vi "LightStrip25.vi"() -> ()   [LabVIEW 2023]
uses:
  <vilib>/Platform/TimedLoop/XDataNode/timing_clust.ctl
  <vilib>/Platform/TimedLoop/XDataNode/nitl_modes.ctl
  <vilib>/Platform/TimedLoop/XDataNode/wakeup.ctl
  <vilib>/platform/TimedLoop/XDataNode/XDataNode.xnode
  <vilib>/Platform/TimedLoop/XDataNode/XDNodeRunTimeDep.lvlib
  BlingLibrary/ArduinoSerialBling.lvlib
panel:
  out "?":string
  in  "Driver color":u32(colorbox)
  in  "Match Ending \"timer\" (s)":dbl(slide) scale=0.0..30.0 scale format="%#_2g"
  in  "Robot State":T1(ring)
  out "LEDs":u32[](array[colorbox])
  in  "?":bool
  # "Light modes:\n\nConnected (default): \"pit mode\"; lights should be off by default during match\n\nDisconnected: flash red when disconnected/disabled?\n\nAutonomous: purple during auto\n\nAlgae: flash teal when running algae intake\n\nCoral: white when running coral intake\n\nOuttaking: flash green when outtaking/scoring\n\nAuto align; brief rainbow when aligning to Apriltag\n\nMatch ending: slowly slide timer to \"simulate\". Blue to red from outside, flash white when match end\n\nDefense: police strobe if/when defending\n\nDriver color: can be set on dashboard"
  # "Light strip"
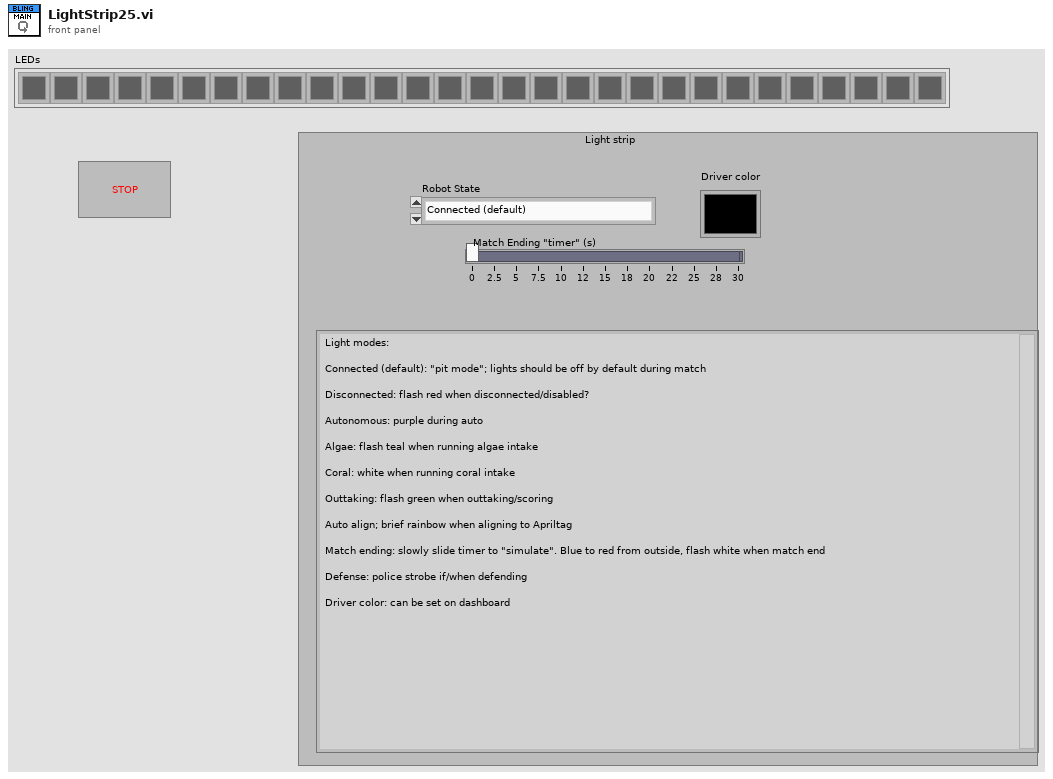
[diagram p1: front panel]
types:
  T1 = enum16{"Connected (default)", "Disconnected", "Autonomous", "Algae intake", "Coral intake", "Outtaking", "Auto align", "Match Ending", "Defense", "Driver Color"}
  T2 = enum16{"Connected (default)", "Disconnected", "Autonomous", "Browning", "Algae", "Coral", "Outtaking", "Auto align", "Match ending", "Defense", "Driver Color"}
  T3 = typedef "ArduinoSerialBling.lvlib/ControlState.ctl" = cluster{"VISA resource name":refnum<visa-resource-name>, "Synchronous":bool, "Value Width":enum16{"4-bit", "8-bit"}, "ChainMask":u8, "Chains":T4[], "OfflineMode":bool}
  T4 = typedef "ArduinoSerialBling.lvlib/ChainState.ctl" = cluster{"ChainNumber":u8, "numLeds":u8, "LED Colors":u32[]}
  T5 = typedef "XDNodeRunTimeDep.lvlib/timing_clust.ctl" = cluster{"Expected End [f-1]":u64, "Actual End [f-1]":u64, "Finished Late? [f-1]":bool, "Expected End [i-1]":u64, "Actual End [i-1]":u64, "Finished Late? [i-1]":bool, "Expected Start [i]":u64, "Actual Start [i]":u64, "Expected Start [f]":u64, "Actual Start [f]":u64, "Source Name":string, "Structure Name":string, "Period":i64, "Deadline":i64, "Offset":i64, "Start":i64, "Priority":i32, "Timeout":i32, "Mode":T6, "Wakeup Reason":T7, "Error":errorcluster, "Source Type":string, "Secondary Source Type":string, "Global End Time":u64, "Global Start Time":u64, "Frame Duration":u64, "Iteration Duration":u64, "Assigned CPU":i32, "I/O Scan Engine Mode":u32}
  T6 = typedef "XDNodeRunTimeDep.lvlib/nitl_modes.ctl" = enum32{"No Change", "Process missed periods, maintain original phase", "Discard missed periods, maintain original phase", "Process missed periods, ignore original phase", "Discard missed periods, ignore original phase"}
  T7 = typedef "XDNodeRunTimeDep.lvlib/wakeup.ctl" = enum32{"Normal", "Aborted", "Asynchronous wakeup", "Timing source error", "Timed loop error", "Timeout"}
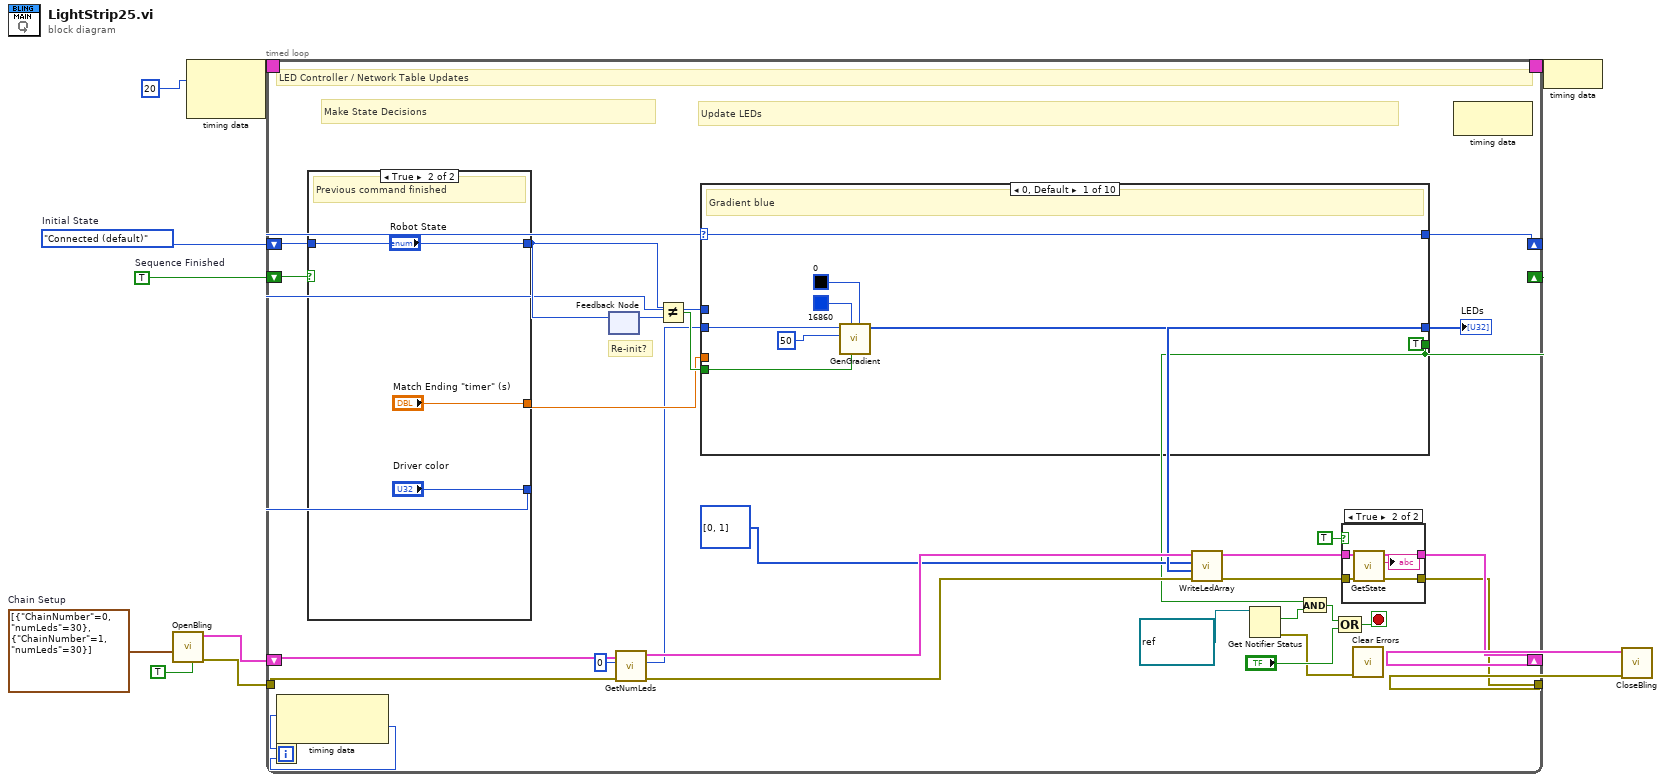
[diagram p0: block diagram]
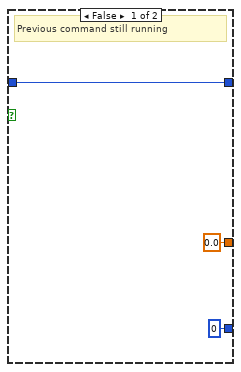
[diagram p3: hidden frame]
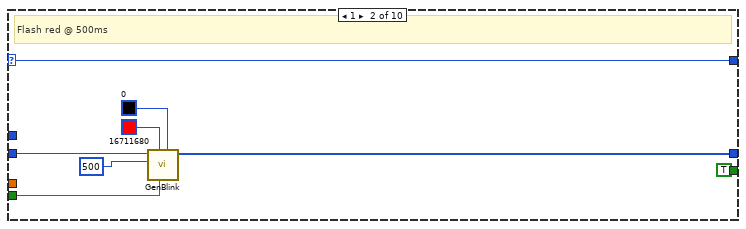
[diagram p4: hidden frame]
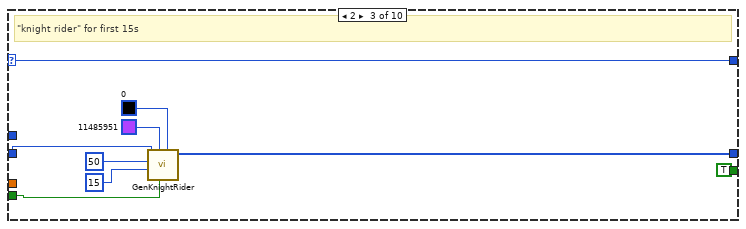
[diagram p5: hidden frame]
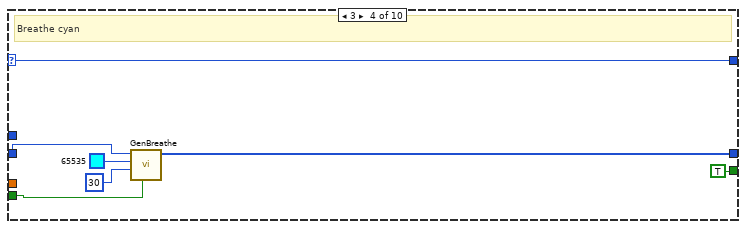
[diagram p6: hidden frame]
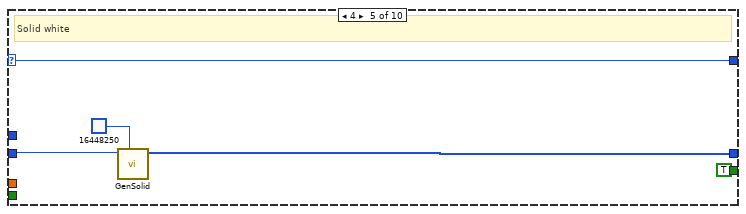
[diagram p7: hidden frame]
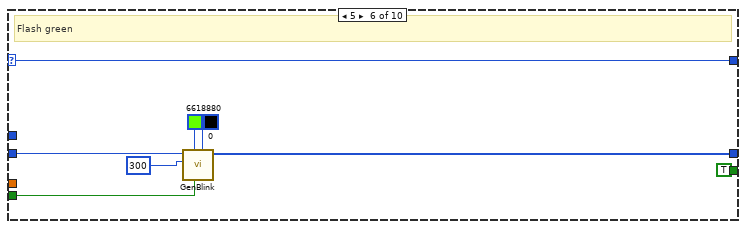
[diagram p8: hidden frame]
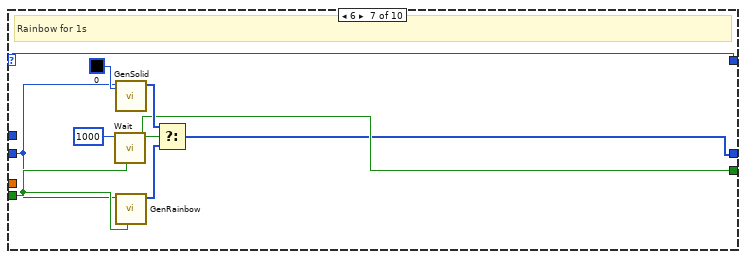
[diagram p9: hidden frame]
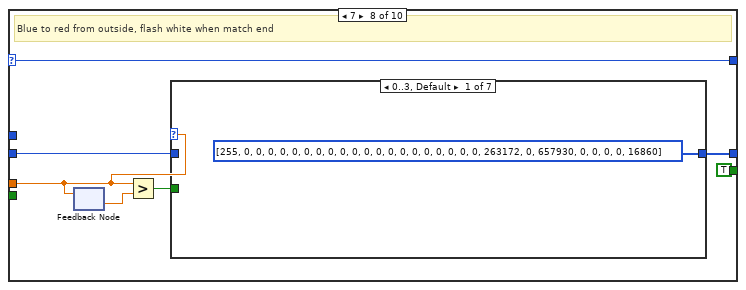
[diagram p10: hidden frame]
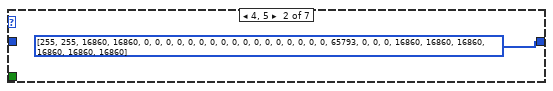
[diagram p11: hidden frame]
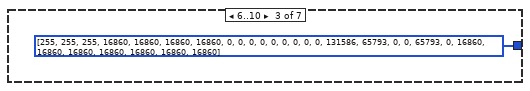
[diagram p12: hidden frame]
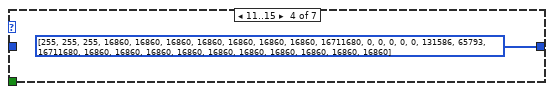
[diagram p13: hidden frame]
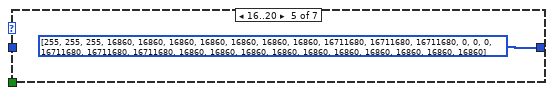
[diagram p14: hidden frame]
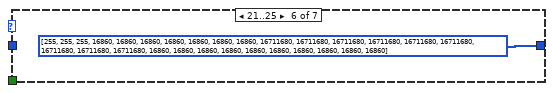
[diagram p15: hidden frame]
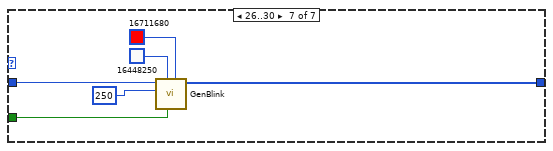
[diagram p16: hidden frame]
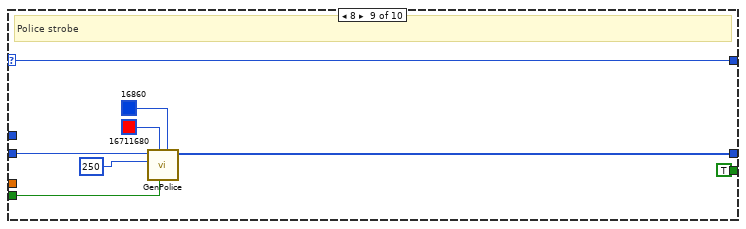
[diagram p17: hidden frame]
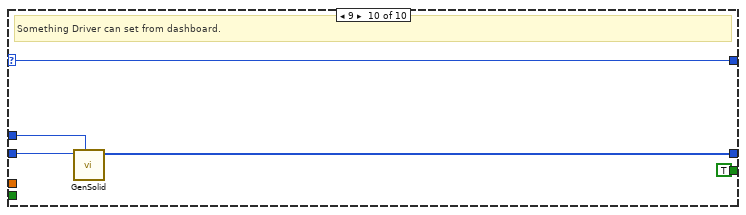
[diagram p18: hidden frame]
diagram:
  w3 = TRUE  # Sequence Finished
  w4 = T2."Connected (default)"  # Initial State
  w8 = cluster{"ChainNumber":u8, "numLeds":u8}[] [{"ChainNumber"=0, "numLeds"=30}, {"ChainNumber"=1, "numLeds"=30}]  # Chain Setup
  n1 = call "OpenBling.vi"("OfflineMode"=TRUE ("Bling Offline Mode"), "Chain Setup"=w8) -> ("error out"=w7:errorcluster, "ControlState"=w1:T3)  [unwired: 8 in]
  n2 = node-c288(i64 20 ("Period")) -> (w11:T5)  [unwired: 1 in]
  n3 = timed-loop {
    timing: w11 -> [_]
    timing-out: [_] -> w10
    tunnel: w7 -> [w34]
    tunnel: [w24] -> w6
    shift-right: [w40] -> _
    shift-left: w4 -> [w38]
    shift-right: [w17] -> _
    shift-left: w3 -> [w39]
    shift-right: [w25] -> w5
    shift-left: w1 -> [w19]
    stop <- w41 stop-if-true
    # "Re-init?"
    # "Update LEDs"
    # "Make State Decisions"
    # "LED Controller / Network Table Updates"
    n4 = node-c288() -> (w21:i64, w20:i64)  [unwired: 1 in]
    n5 = Subtract(x=w21, y=w20) -> ()  [unwired: 1 out]
    n6 = case shown="True" w39 {
      tunnel: [w51 "Robot State"] -> w36
      tunnel: w38 -> [w51 _]
      tunnel: [0.0 "Match Ending \"timer\" (s)"] -> w30
      tunnel: [u32 0 "Driver color"] -> w29
      frame False {
        # "Previous command still running"
      }
      frame True {
        # "Previous command finished"
      }
    }
    n7 = feedback-in #1(w36) -> ()
    n8 = feedback #1() -> (w37:u16)  [unwired: 1 in]
    n9 = call "GetNumLeds.vi"("error in (no error)"=w34, "Chain"=0, "ControlState"=w19) -> ("error out"=w31:errorcluster, "NumLeds"=w26:i32, "ControlState 2"=w32:T3)  [unwired: 6 in]
    n10 = Not Equal?(x=w36, y=w37) -> (x != y?=w35:bool)
    n11 = case shown="0, Default" w36 {
      selector: w36 -> [w61 w70 w78 w85 w90 w98 w108 w115 w134 w137]
      tunnel: [w61 w70 w78 w85 w90 w98 w108 w115 w134 w137] -> w40
      tunnel: [TRUE TRUE TRUE TRUE TRUE TRUE w101 TRUE TRUE TRUE] -> w17
      tunnel: w35 -> [w56 w63 w71 w84 _ w93 w106 _ w131 _]
      tunnel: w26 -> [w60 w64 w77 w83 w88 w94 w102 w112 w133 w139]
      tunnel: [w57 w68 w72 w80 w87 w92 w100 w113 w130 w138] -> w28
      tunnel: w30 -> [_ _ _ _ _ _ _ w110 _ _]
      tunnel: w29 -> [_ _ _ _ _ _ _ _ _ w136]
      frame 0, Default {
        # "Gradient blue"
        n12 = call "GenGradient.vi"("Color 2"=u32 0, "Reset"=w56, "Color 1"=u32 16860, "Sine Rate"=50, "NumLeds"=w60) -> ("LED Array"=w57:u32[])  [unwired: 6 in]
      }
      frame 1 {
        # "Flash red @ 500ms"
        n13 = call "GenBlink.vi"("Color 2"=u32 0, "Reset"=w63, "Color 1"=u32 16711680, "Period (ms)"=500, "NumLeds"=w64) -> ("Array"=w68:u32[])  [unwired: 5 in, 1 out]
      }
      frame 2 {
        # "\"knight rider\" for first 15s"
        n14 = call "GenKnightRider.vi"("Background Color"=u32 0, "Reset"=w71, "Foreground Color"=u32 11485951, "Blending LEDs"=u8 15, "Sine Rate"=50, "NumLeds"=w77) -> ("Array"=w72:u32[])  [unwired: 4 in, 1 out]
      }
      frame 3 {
        # "Breathe cyan"
        n15 = call "GenBreathe.vi"("Reset"=w84, "Sine Rate"=30, "Color Box"=u32 65535, "NumLeds"=w83) -> ("Array"=w80:u32[])  [unwired: 6 in, 1 out]
      }
      frame 4 {
        # "Solid white"
        n16 = call "GenSolid.vi"("Color"=u32 16448250, "NumLeds"=w88) -> ("Array"=w87:u32[])  [unwired: 9 in]
      }
      frame 5 {
        # "Flash green"
        n17 = call "GenBlink.vi"("Color 2"=u32 0, "Reset"=w93, "Color 1"=u32 6618880, "Period (ms)"=300, "NumLeds"=w94) -> ("Array"=w92:u32[])  [unwired: 5 in, 1 out]
      }
      frame 6 {
        # "Rainbow for 1s"
        n18 = call "Wait.vi"("Reset"=w106, "milliseconds to wait"=1000) -> ("Finished"=w101:bool)  [unwired: 9 in]
        n19 = call "GenSolid.vi"("Color"=u32 0 ("Color 2"), "NumLeds"=w102) -> ("Array"=w104:u32[])  [unwired: 9 in]
        n20 = call "GenRainbow.vi"("Reset"=w106, "NumLeds"=w102) -> ("Rainbow"=w103:u32[])  [unwired: 9 in]
        n21 = Select(t=w104, s=w101, f=w103) -> (s? t:f=w100:u32[])
      }
      frame 7 {
        # "Blue to red from outside, flash white when match end"
        n22 = feedback-in #2(w110) -> ()
        n23 = feedback #2() -> (w111:dbl)  [unwired: 1 in]
        n24 = Greater?(x=w110, y=w111) -> (0:w109:bool)
        n25 = case shown="0..3, Default" w110 {
          tunnel: [u32[] [255, 0, 0, 0, 0, 0, 0, 0, 0, 0, 0, 0, 0, 0, 0, 0, 0, 0, 0, 0, 0, 263172, 0, 657930, 0, 0, 0, 0, 16860] u32[] [255, 255, 16860, 16860, 0, 0, 0, 0, 0, 0, 0, 0, 0, 0, 0, 0, 0, 0, 0, 0, 0, 65793, 0, 0, 0, 16860, 16860, 16860, 16860, 16860, 16860] u32[] [255, 255, 255, 16860, 16860, 16860, 16860, 0, 0, 0, 0, 0, 0, 0, 0, 0, 131586, 65793, 0, 0, 65793, 0, 16860, 16860, 16860, 16860, 16860, 16860, 16860] u32[] [255, 255, 255, 16860, 16860, 16860, 16860, 16860, 16860, 16860, 16711680, 0, 0, 0, 0, 0, 131586, 65793, 16711680, 16860, 16860, 16860, 16860, 16860, 16860, 16860, 16860, 16860, 16860] u32[] [255, 255, 255, 16860, 16860, 16860, 16860, 16860, 16860, 16860, 16711680, 16711680, 16711680, 0, 0, 0, 16711680, 16711680, 16711680, 16860, 16860, 16860, 16860, 16860, 16860, 16860, 16860, 16860, 16860] u32[] [255, 255, 255, 16860, 16860, 16860, 16860, 16860, 16860, 16860, 16711680, 16711680, 16711680, 16711680, 16711680, 16711680, 16711680, 16711680, 16711680, 16860, 16860, 16860, 16860, 16860, 16860, 16860, 16860, 16860, 16860] w122] -> w113
          tunnel: w112 -> [_ _ _ _ _ _ w127]
          tunnel: w109 -> [_ _ _ _ _ _ w123]
          frame 0..3, Default {
          }
          frame 4, 5 {
          }
          frame 6..10 {
          }
          frame 11..15 {
          }
          frame 16..20 {
          }
          frame 21..25 {
          }
          frame 26..30 {
            n26 = call "GenBlink.vi"("Color 2"=u32 16711680, "Reset"=w123, "Color 1"=u32 16448250, "Period (ms)"=250, "NumLeds"=w127) -> ("Array"=w122:u32[])  [unwired: 5 in, 1 out]
          }
        }
      }
      frame 8 {
        # "Police strobe"
        n27 = call "GenPolice.vi"("Color 2"=u32 16860, "Reset"=w131, "Color 1"=u32 16711680, "Period"=250, "NumLeds"=w133) -> ("Array"=w130:u32[])  [unwired: 6 in]
      }
      frame 9 {
        # "Something Driver can set from dashboard."
        n28 = call "GenSolid.vi"("Color"=w136, "NumLeds"=w139) -> ("Array"=w138:u32[])  [unwired: 9 in]
      }
    }
    "LEDs" <- w28
    n29 = call "WriteLedArray.vi"("error in (no error)"=w31, "LED Colors"=w28, "Chains"=u8[] [0, 1], "ControlState in"=w32) -> ("error out"=w22:errorcluster, "ControlState out"=w23:T3)  [unwired: 5 in, 1 out]
    n30 = Get Notifier Status(notifier=refnum<notifier> refnum ("Cancel Ref")) -> (current notification=w18:bool, error out=w13:errorcluster)  [unwired: 1 in, 3 out]
    n31 = And(x=w17, y=w18) -> (x .and. y?=w16:bool)
    n32 = Compound Arithmetic op=OR(w16, "?") -> (w41:bool)
    n33 = case shown="True" TRUE {
      tunnel: [w43 w48] -> w25
      tunnel: [w42 w47] -> w24
      tunnel: w23 -> [w43 w45]
      tunnel: w22 -> [w42 w44]
      frame False {
      }
      frame True {
        n34 = call "GetState.vi"("error in (no error)"=w44, "ControlState in"=w45) -> ("error out"=w47:errorcluster, "State"=→"?":string, "ControlState out"=w48:T3)  [unwired: 7 in]
      }
    }
    n35 = call <vilib>:"Clear Errors.vi"("error in (no error)"=w13) -> ()  [unwired: 5 in, 2 out]
    n36 = node-c288() -> ()  [unwired: 1 in, 1 out]
  }
  n37 = node-c288(w10) -> ()
  n38 = call "CloseBling.vi"("error in (no error)"=w6, "ControlState in"=w5) -> ()  [unwired: 9 in, 1 out]
